vi "init TVDisplay Ctr Color.vi"(8 "error in (no error)":errorcluster, 10 "Ctr Color":cluster{"Label":string, "Color":u32}[](array[cluster]), 11 "appended array":refnum<vi>[](array[refnum])) -> (0 "error out":errorcluster)   [LabVIEW 2014]
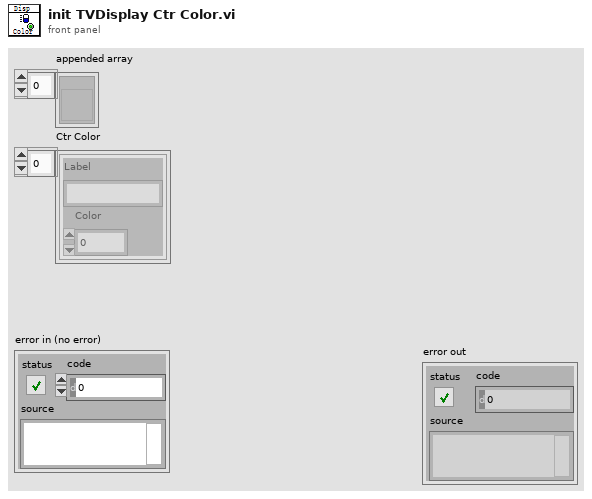
[diagram p1: front panel]
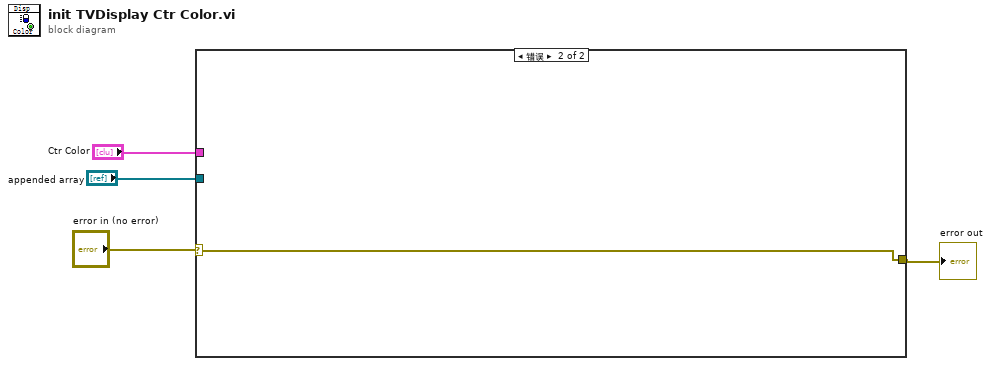
[diagram p0: block diagram]
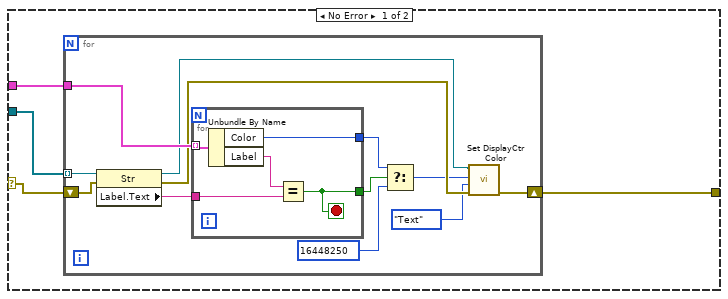
[diagram p2: hidden frame]
diagram:
  n1 = case shown="错误" "error in (no error)" {
    selector: "error in (no error)" -> [w8 w26]
    tunnel: "appended array" -> [w7 _]
    tunnel: "Ctr Color" -> [w6 _]
    tunnel: [w5 w26] -> w1
    frame No Error {
      n2 = for {
        tunnel: w7 -> [w19] mode=indexing
        tunnel: w6 -> [w18]
        shift-right: [w9] -> w5
        shift-left: w8 -> [w20]
        n3 = property class="Str"(reference=w19, error in=w20) -> (reference out=w16:refnum<vi>, error out=w15:errorcluster, "Label.Text"=w17:string)
        n4 = for {
          tunnel: w18 -> [w25] mode=indexing
          tunnel: w17 -> [w24]
          tunnel: [w22] -> w13
          tunnel: [w21] -> w14
          stop <- w21 stop-if-true
          n5 = Unbundle By Name(w25) -> ("Color"=w22:u32, "Label"=w23:string)
          n6 = Equal?(x=w23, y=w24) -> (x = y?=w21:bool)
        }
        n7 = Select(t=w13, s=w14, f=16448250) -> (s? t:f=w11:u32)
        n8 = call "Set DisplayCtr Color.vi"("error in (no error)"=w15, "Mode"=enum16{"Label", "Caption", "Text"}."Text", "Color Box"=w11, "Ctr Ref"=w16) -> ("error IO"=w9:errorcluster)  [unwired: 7 in]
      }
    }
    frame Error {
    }
  }
  "error out" <- w1
